vi "random-dice.vi"   [LabVIEW 2012]
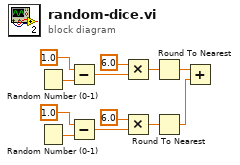
[diagram p0: block diagram]
diagram:
  n1 = Random Number (0-1)() -> (number: 0 to 1=w11:dbl)
  n2 = Random Number (0-1)() -> (number: 0 to 1=w6:dbl)
  n3 = Subtract(x=1.0, y=w11) -> (x-y=w9:dbl)
  n4 = Subtract(x=1.0, y=w6) -> (x-y=w4:dbl)
  n5 = Multiply(x=6.0, y=w9) -> (x*y=w8:dbl)
  n6 = Multiply(x=6.0, y=w4) -> (x*y=w3:dbl)
  n7 = Round To Nearest(number=w8) -> (nearest integer value=w1:dbl)
  n8 = Round To Nearest(number=w3) -> (nearest integer value=w2:dbl)
  n9 = Add(x=w1, y=w2) -> ()  [unwired: 1 out]
